vi "Check for Clock Fault.vi"(8 "error in":errorcluster, 11 "refnum in":refnum<k20>) -> (0 "error out":errorcluster, 3 "refnum out":refnum<k20>)   [LabVIEW 2021, in "Device Session.lvclass"]
uses:
  Device Session.lvclass
  <vilib>/FPGAPlugInAG/Dynamic/niLvFpga_Download_Dynamic.vi
  <vilib>/FPGAPlugInAG/Dynamic/niLvFpga_Run_Dynamic.vi
  <vilib>/rvi/interface/nirviMethod/nirviMethod.xnode
  <instrlib>/HSAI-RIO/Config/Group A/v1/Host/Main/niHSAI Group A Config v1 Host.lvclass
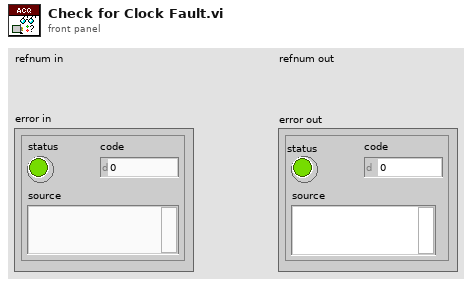
[diagram p1: front panel]
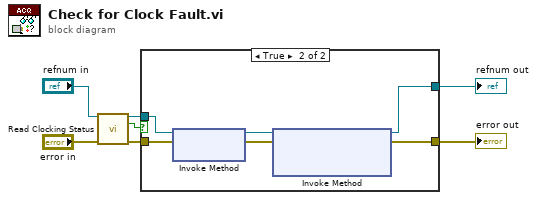
[diagram p0: block diagram]
diagram:
  n1 = call <instrlib>:"Read Clocking Status.vi"("fpga interface in"="refnum in", "error in"="error in") -> ("fpga interface out"=w3:refnum<k20>, "clock fault?"=w5:bool, "error out"=w4:errorcluster)  [unwired: 11 in]
  n2 = case shown="True" w5 {
    tunnel: w4 -> [w9 w13]
    tunnel: [w9 w12] -> w2
    tunnel: [w8 w10] -> w7
    tunnel: w3 -> [w8 w11]
    frame False {
    }
    frame True {
      n3 = xnode "Invoke Method"("FPGA VI Reference In"=w11, "error in"=w13) -> ("FPGA VI Reference Out"=w14:refnum<k20>, "error out"=w15:errorcluster)
      n4 = xnode "Invoke Method"("FPGA VI Reference In"=w14, "error in"=w15) -> ("FPGA VI Reference Out"=w10:refnum<k20>, "error out"=w12:errorcluster)  [unwired: 1 in]
    }
  }
  "refnum out" <- w7
  "error out" <- w2
